vi "Replace text in error.vi"(0 "Text to find":string, 5 "Replace with":string, 11 "error in (no error)":errorcluster) -> (15 "error out":errorcluster)   [LabVIEW 2020]
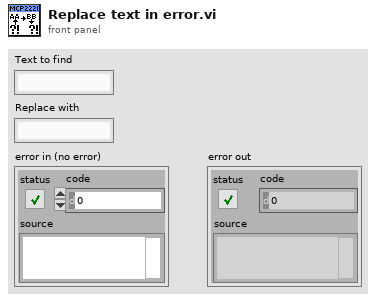
[diagram p1: front panel]
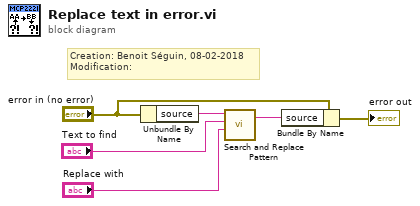
[diagram p0: block diagram]
diagram:
  # "Creation: Benoit Séguin, 08-02-2018\nModification:"
  n1 = Unbundle By Name("error in (no error)") -> ("source"=w6:string)
  n2 = call <vilib>:"Search and Replace Pattern.vi"("string"=w6, "regular expression (\"\")"="Text to find", "replace string (\"\")"="Replace with") -> ("result string"=w2:string)  [unwired: 2 in, 1 out]
  n3 = Bundle By Name(cluster="error in (no error)", "source"=w2) -> (→"error out":errorcluster)
